vi "Read Player Info.vi"(8 "error in (no error)":errorcluster, 11 "Runner in":refnum<class "Runner.lvclass">) -> (0 "error out":errorcluster, 2 "Player Info":T1={"Name"="", "Color Box"=0, "Gloat Phrase"="All your base are belong to us!!"}, 3 "Runner out":refnum<class "Runner.lvclass">)   [LabVIEW 2014, in "Runner.lvclass"]
uses:
  Runner.lvclass
  Player Info.ctl
  Runner.lvclass/Runner.ctl
  SquareBattle.lvclass
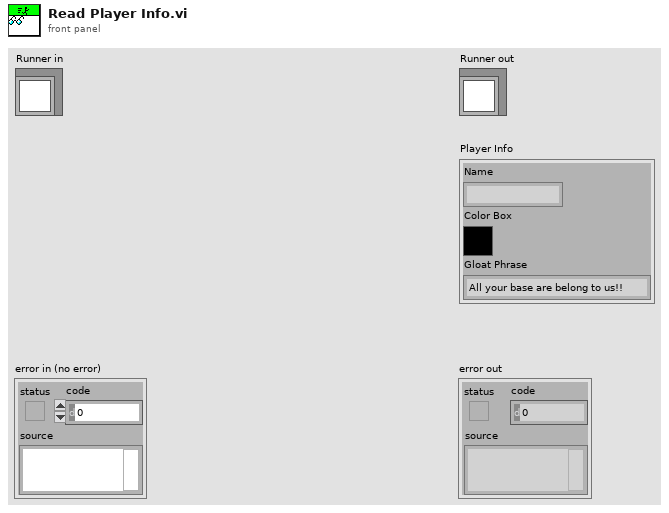
[diagram p1: front panel]
types:
  T1 = typedef "SquareBattle.lvclass/Player Info.ctl" = cluster{"Name":string, "Color Box":u32, "Gloat Phrase":string}
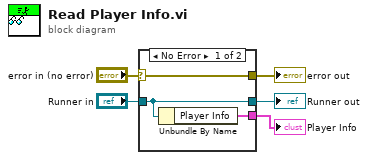
[diagram p0: block diagram]
diagram:
  n1 = case shown="No Error" "error in (no error)" {
    selector: "error in (no error)" -> [w8 w9]
    tunnel: [w8 w9] -> w4
    tunnel: [w7 w10] -> w2
    tunnel: "Runner in" -> [w7 w10]
    tunnel: [w6 _] -> w1
    frame No Error {
      n2 = Unbundle By Name(w7) -> ("Player Info"=w6:T1)
    }
    frame Error {
    }
  }
  "error out" <- w4
  "Runner out" <- w2
  "Player Info" <- w1
